vi "Translator.File.Read.Msg.vi"(8 "error in":errorcluster, 10 "Translation folder":path=path "D:/PL_0125_Sapphire_Automation_branches/SOFTWARE_v1.1-Translation/settings/Translation-Chinese.ini") -> (0 "error out":errorcluster)   [LabVIEW 2019, in "Tools.lvlib"]
uses:
  Tools.lvlib
  Translator.Enums.ctl
  Translator.Messages.Status.ctl
  Translator.File.MatchStrings (Array).vi
  <vilib>/Utility/config.llb/NI_LVConfig.lvlib
panel:
  out "#old":i32[](array[numeric])
  out "#new":i32[](array[numeric])
  in  "Enums":T1={"Enum"=enum."b"}
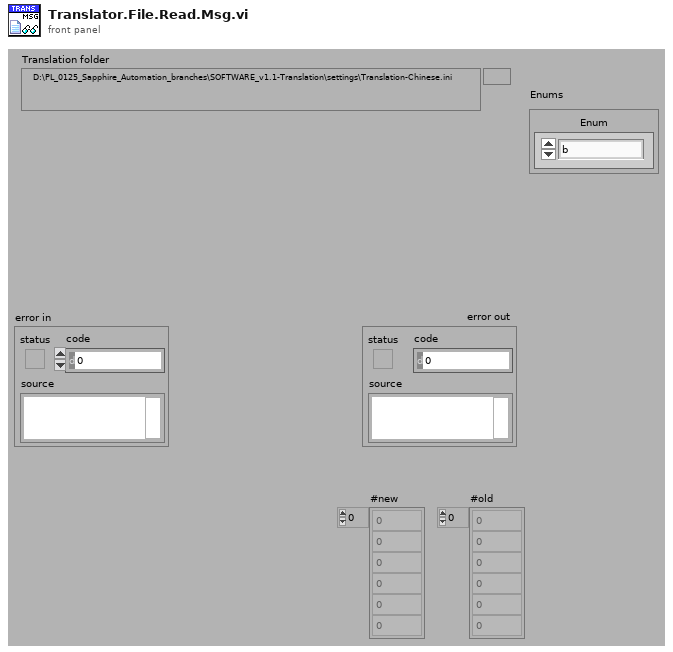
[diagram p1: front panel]
types:
  T1 = typedef "Tools.lvlib/Translator.Enums.ctl" = cluster{"Enum":enum16{"a", "b", "c"}}
  T2 = typedef "Tools.lvlib/Translator.Messages.Status.ctl" = enum16{"-", "Initializing...", "Quitting...", "Close the application?", "Log out?", "System", "All", "IDLE", "Translating...%s", "Restart is required to translate the application! Do you want to restart the PC?", "Restart cancelled. Be aware that some controls may not be fully translated until you restart the application.", "New version available!", "The software is up-to-date", "PC software will be updated after rebooting the PC. Do you want to reboot now?", "RT software will be updated. Make sure that no process is running. Do you want to reboot RT now?", "Updating RT firmware. Please wait...", "Update failed: %s", "Rebooting...", "Rebooting RT. Please wait...", "RT updated to version %s", "Timeout error during update. Check if RT is working", "Closing stations...", "Closing camera interface...", "Closing data acquisition interface...", "Service Option not available in this station!"}
  T3 = typedef "NI_LVConfig.lvlib/Config Data RefNum.ctl" = refnum<k1>
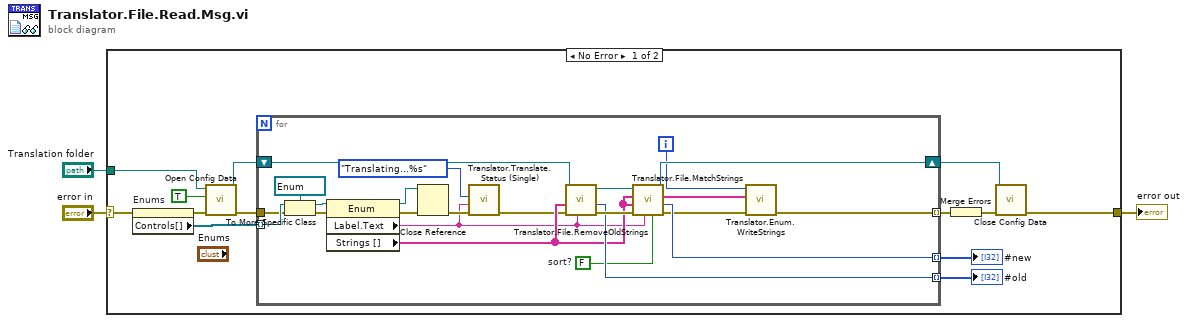
[diagram p0: block diagram]
diagram:
  n1 = case shown="No Error" "error in" {
    selector: "error in" -> [w12 w40]
    tunnel: "Translation folder" -> [w9 _]
    tunnel: [w10 w40] -> w2
    frame No Error {
      n2 = property on="Enums" class="Clust (strict)"(error in=w12) -> (error out=w11:errorcluster, "Controls[]"=w5:refnum<vi>[])  [unwired: 1 in, 1 out]
      n3 = call <vilib>:"Open Config Data.vi"("error in (no error)"=w11, "create file if necessary (T)"=TRUE, "configuration file path"=w9) -> ("error out"=w14:errorcluster, "refnum"=w7:T3)  [unwired: 6 in, 1 out]
      n4 = for {
        tunnel: w5 -> [w39] mode=indexing
        shift-right: [w28] -> w6
        shift-left: w7 -> [w32]
        tunnel: [w27] -> w13 mode=indexing
        tunnel: [w29] -> w8 mode=indexing
        tunnel: w14 -> [w35]
        tunnel: [w18] -> w15 mode=indexing
        i -> [w19]
        w17 = FALSE  # sort?
        n5 = To More Specific Class(target class=refnum<vi> refnum ("reference out"), reference=w39, error in=w35) -> (specific class reference=w38:refnum<vi>, error out=w37:errorcluster)
        n6 = property class="Enum"(reference=w38, error in=w37) -> (reference out=w33:refnum<vi>, error out=w34:errorcluster, "Label.Text"=w22:string, "Strings []"=w26:string[])
        n7 = Close Reference(reference=w33, error in (no error)=w34) -> (error out=w25:errorcluster)
        n8 = call "Translator.Translate.Status (Single).vi"("error in (no error)"=w25, "Arg"=w22, "Msg"=Translator.Messages.Status."Translating...%s" ("msg")) -> ("error out"=w24:errorcluster)  [unwired: 7 in, 1 out]
        n9 = call "Translator.File.RemoveOldStrings.vi"("group"=w22, "error in"=w24, "labels"=w26, "refnum in"=w32) -> ("error out"=w31:errorcluster, "#removed"=w29:i32, "refnum out"=w30:T3)  [unwired: 5 in]
        n10 = call-poly "Translator.File.MatchStrings.vi"("sort? (T)"=w17, "group"=w22, "error in"=w31, "labels"=w26, "default values"=w26, "refnum in"=w30) -> ("error out"=w21:errorcluster, "#added"=w27:i32, "values out"=w20:string[], "refnum out"=w28:T3)  [unwired: 2 in]
        n11 = call "Translator.Enum.WriteStrings.vi"("error out"=w21, "Strings"=w20, "idx"=w19) -> ("error out 2"=w18:errorcluster)  [unwired: 8 in]
      }
      "#new" <- w13
      "#old" <- w8
      n12 = Merge Errors(w15) -> (w4:errorcluster)
      n13 = call <vilib>:"Close Config Data.vi"("error in (no error)"=w4, "refnum"=w6) -> ("error out"=w10:errorcluster)  [unwired: 8 in, 1 out]
    }
    frame Error {
    }
  }
  "error out" <- w2
